vi "Remove dots from file names.vi"(8 "error in (no error)":errorcluster, 11 "file with path":path) -> (0 "error out":errorcluster, 2 "Updated file with no . before extention":string, 3 "dup file with path":path)   [LabVIEW 2011]
doc: "Use this VI to remove the all . out of a file name other then the one marking the extention. Use the return dots after done to restore original file name."
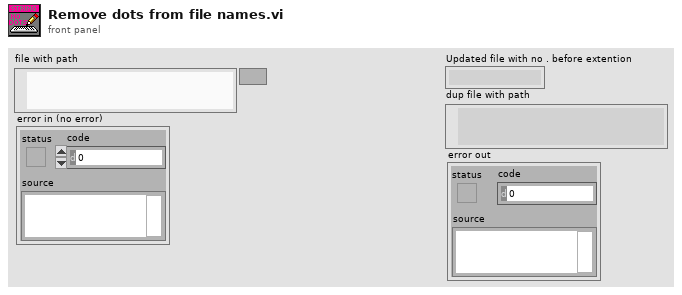
[diagram p1: front panel]
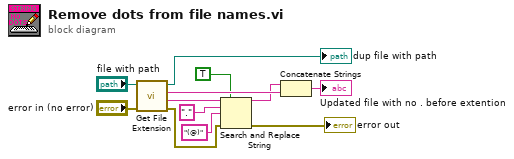
[diagram p0: block diagram]
diagram:
  n1 = call <vilib>:"Get File Extension.vi"("error in (no error)"="error in (no error)", "file"="file with path") -> ("error out"=w10:errorcluster, "filename without extension"=w6:string, "lowercase file extension"=w12:string, "dup file"=→"dup file with path":path)  [unwired: 6 in]
  n2 = Search and Replace String(replace all?=TRUE ("replace all? (F)"), input string=w6, search string=".", replace string="(@)" ("replace string (\"\")"), error in=w10) -> (result string=w11:string, error out=→"error out":errorcluster)  [unwired: 3 in, 2 out]
  n3 = Concatenate Strings(w11, w12) -> (→"Updated file with no . before extention":string)
